vi "XYGraph_appearance.vi"() -> ()   [LabVIEW 2020]
panel:
  in  "Index Cluster":i32
  out "Array of DUT Cluster":cluster{"DUT (x)":dbl[], "DUT (y)":dbl[]}[](array[cluster])
  out "XY Graph":cluster{"DUT (x)":dbl[], "DUT (y)":dbl[]}[](graph)
  out "Display -> REFNUM : Test Voltages Results Temp Array":dbl[](array[numeric])
  out "Display -> REFNUM : Capacitance Results Temp Array":dbl[](array[numeric])
  in  "Array Size":i32
  out "Display -> GLOBAL VARIABLE : Array size(s)":i32
  in  "Test Voltages Results Temp Array":dbl[](array[numeric])
  in  "Capacitance Results Temp Array":dbl[](array[numeric])
  out "error out":errorcluster
  in  "error in (no error)":errorcluster
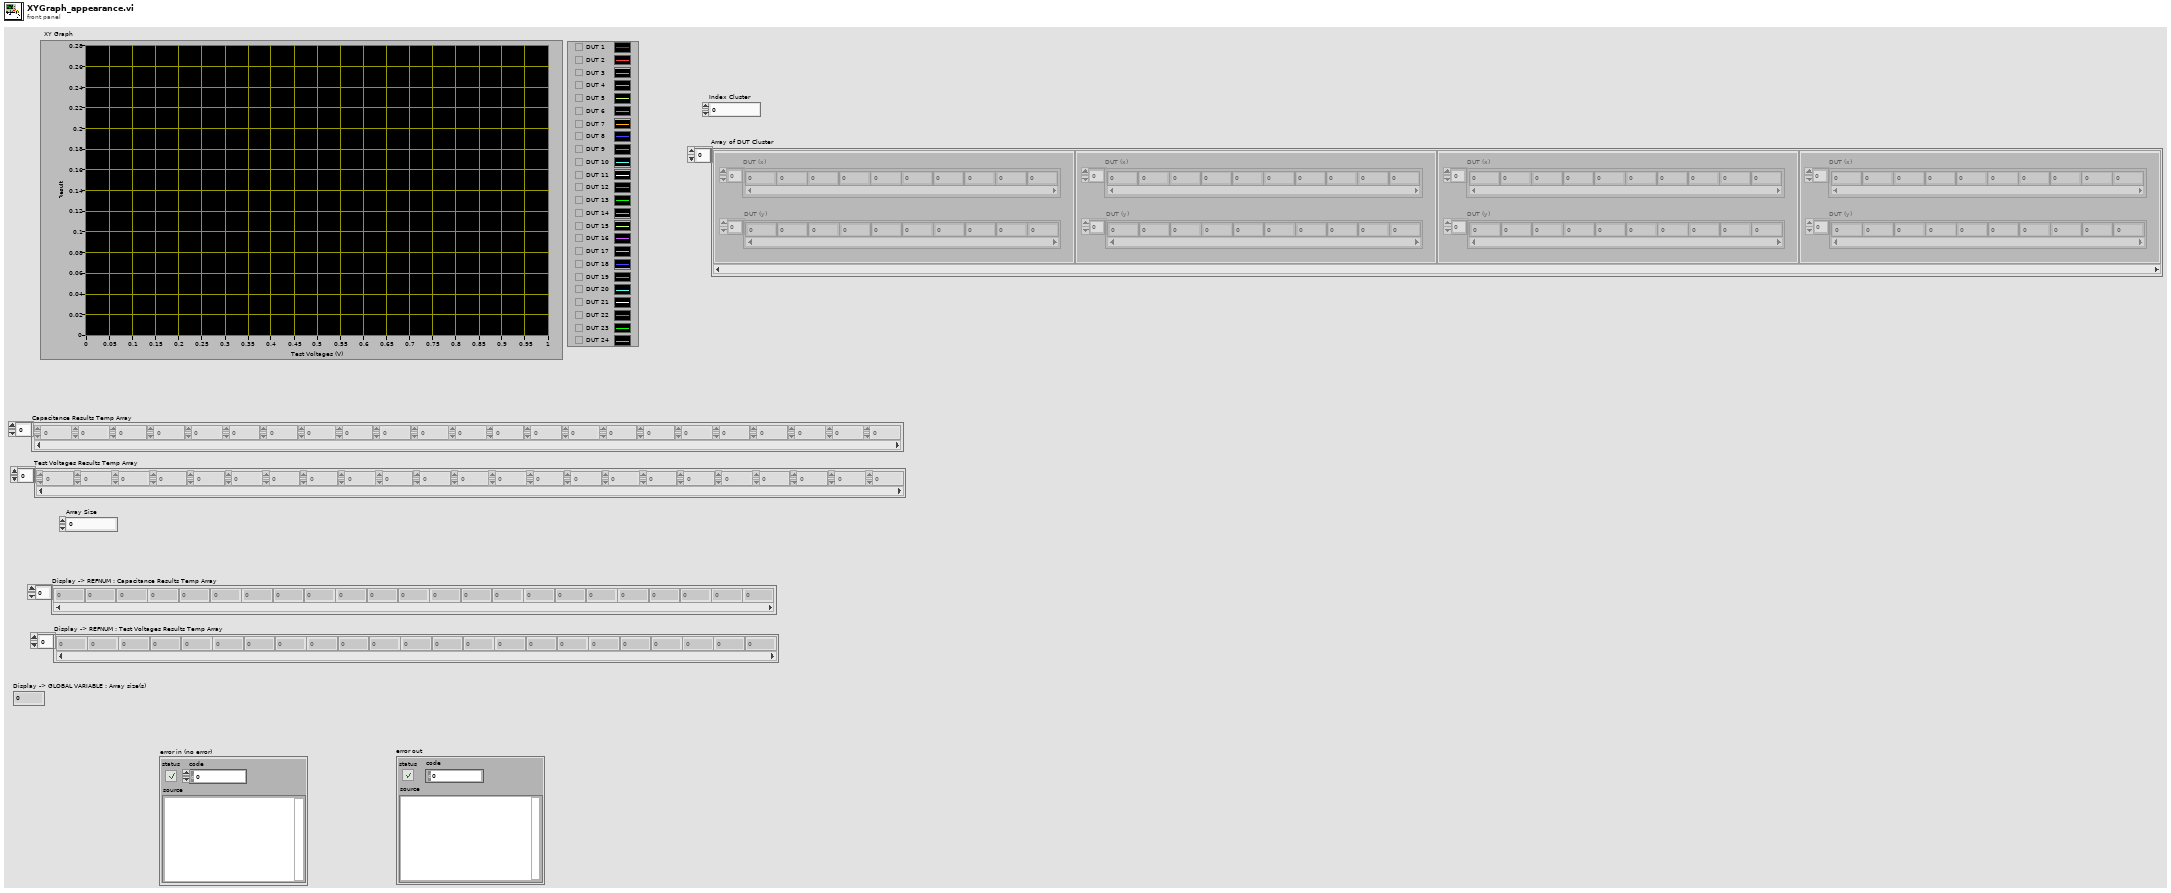
[diagram p1: front panel]
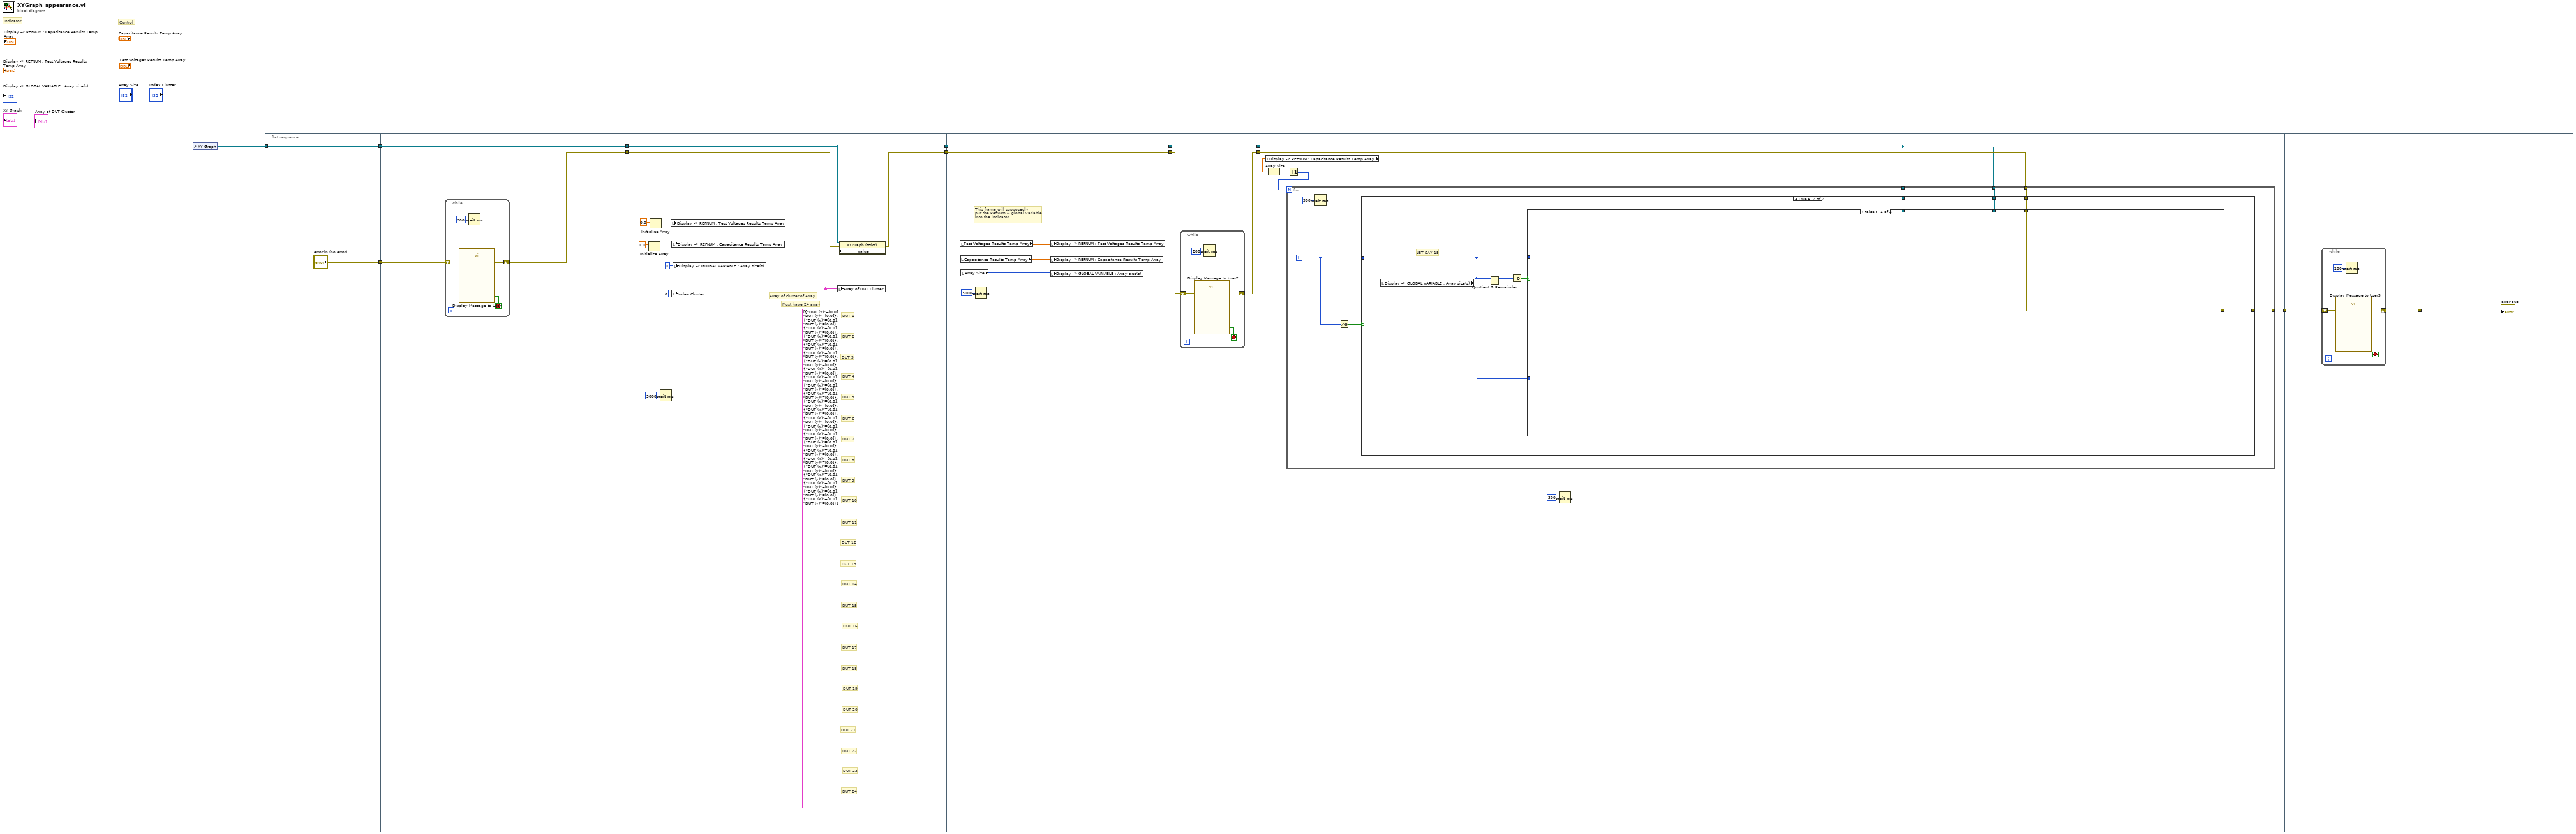
[diagram p0: block diagram]
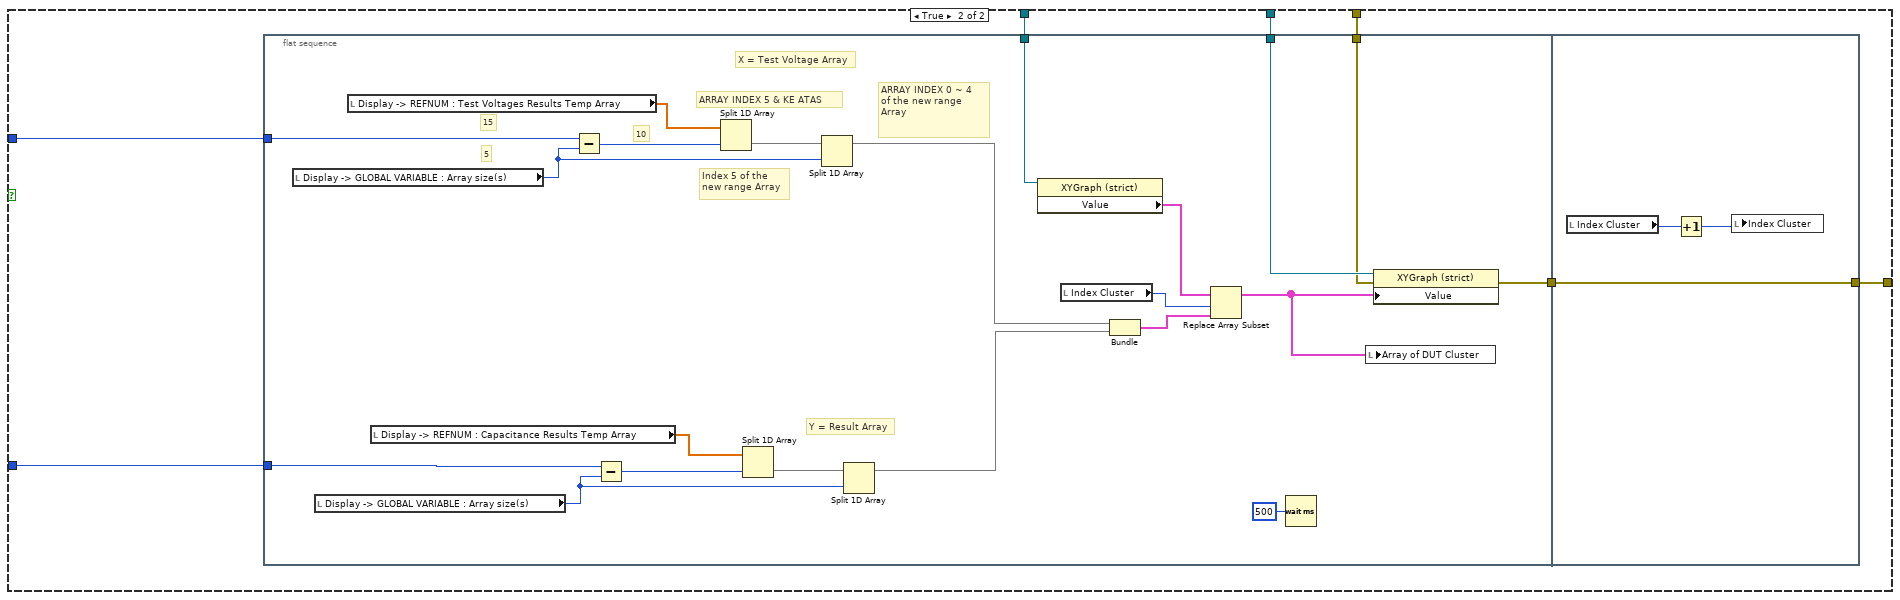
[diagram p3: hidden frame]
diagram:
  # "Indicator"
  # "Control"
  n1 = control-ref of="XY Graph"() -> (w1:refnum<vi>)
  n2 = flat-sequence {
    tunnel: w1 -> [w15]
    tunnel: [w15] -> w13
    tunnel: ["error in (no error)"] -> w12
    tunnel: [w18] -> w11
    tunnel: [w17] -> w10
    tunnel: w13 -> [w18]
    tunnel: w12 -> [w16]
    tunnel: [w27] -> w9
    tunnel: w11 -> [w27]
    tunnel: [w25] -> w8
    tunnel: w10 -> [w26]
    tunnel: [w35] -> w7
    tunnel: w9 -> [w35]
    tunnel: [w34] -> w6
    tunnel: w8 -> [w34]
    tunnel: [w42] -> w5
    tunnel: w7 -> [w42]
    tunnel: [w40] -> w4
    tunnel: w6 -> [w41]
    tunnel: w5 -> [w49]
    tunnel: w4 -> [w51]
    tunnel: [w50] -> w3
    tunnel: w3 -> [w103]
    tunnel: [w102] -> w2
    tunnel: w2 -> [w108]
    frame #0 {
    }
    frame #1 {
      n3 = while {
        shift-right: [w20] -> w17
        shift-left: w16 -> [w21]
        stop <- w19 stop-if-true
        n4 = call "Display Message to User"("error in (no error)"=w21) -> ("error out"=w20:errorcluster, "OK"=w19:bool)  [unwired: 9 in]
        n5 = Wait (ms)(milliseconds to wait=u32 200) -> ()  [unwired: 1 out]
      }
    }
    frame #2 {
      w24 = cluster{"DUT (x)":dbl[], "DUT (y)":dbl[]}[] [{"DUT (x)"=[0.0], "DUT (y)"=[0.0]}, {"DUT (x)"=[0.0], "DUT (y)"=[0.0]}, {"DUT (x)"=[0.0], "DUT (y)"=[0.0]}, {"DUT (x)"=[0.0], "DUT (y)"=[0.0]}, {"DUT (x)"=[0.0], "DUT (y)"=[0.0]}, {"DUT (x)"=[0.0], "DUT (y)"=[0.0]}, {"DUT (x)"=[0.0], "DUT (y)"=[0.0]}, {"DUT (x)"=[0.0], "DUT (y)"=[0.0]}, {"DUT (x)"=[0.0], "DUT (y)"=[0.0]}, {"DUT (x)"=[0.0], "DUT (y)"=[0.0]}, {"DUT (x)"=[0.0], "DUT (y)"=[0.0]}, {"DUT (x)"=[0.0], "DUT (y)"=[0.0]}, {"DUT (x)"=[0.0], "DUT (y)"=[0.0]}, {"DUT (x)"=[0.0], "DUT (y)"=[0.0]}, {"DUT (x)"=[0.0], "DUT (y)"=[0.0]}, {"DUT (x)"=[0.0], "DUT (y)"=[0.0]}, {"DUT (x)"=[0.0], "DUT (y)"=[0.0]}, {"DUT (x)"=[0.0], "DUT (y)"=[0.0]}, {"DUT (x)"=[0.0], "DUT (y)"=[0.0]}, {"DUT (x)"=[0.0], "DUT (y)"=[0.0]}, {"DUT (x)"=[0.0], "DUT (y)"=[0.0]}, {"DUT (x)"=[0.0], "DUT (y)"=[0.0]}, {"DUT (x)"=[0.0], "DUT (y)"=[0.0]}, {"DUT (x)"=[0.0], "DUT (y)"=[0.0]}] ("Array of DUT Cluster")
      # "DUT 24"
      # "DUT 23"
      # "DUT 22"
      # "DUT 21"
      # "DUT 20"
      # "DUT 19"
      # "DUT 18"
      # "DUT 17"
      # "DUT 16"
      # "DUT 15"
      # "DUT 14"
      # "DUT 13"
      # "DUT 12"
      # "DUT 11"
      # "DUT 10"
      # "DUT 9"
      # "DUT 8"
      # "DUT 7"
      # "DUT 6"
      # "DUT 5"
      # "DUT 4"
      # "DUT 3"
      # "DUT 2"
      # "DUT 1"
      # "Array of cluster of Array"
      # "Must have 24 array"
      n6 = Initialize Array(0.0 ("element")) -> (w29:dbl[])  [unwired: 1 in]
      n7 = Initialize Array(0.0 ("element")) -> (w30:dbl[])  [unwired: 1 in]
      n8 = Wait (ms)(milliseconds to wait=u32 3000) -> ()  [unwired: 1 out]
      n9 = local write "Display -> REFNUM : Test Voltages Results Temp Array"(w30) -> ()
      n10 = local write "Display -> REFNUM : Capacitance Results Temp Array"(w29) -> ()
      n11 = local write "Index Cluster"(0 ("Index Cluster")) -> ()
      n12 = local write "Display -> GLOBAL VARIABLE : Array size(s)"(0 ("Display -> GLOBAL VARIABLE : Array size(s)")) -> ()
      n13 = local write "Array of DUT Cluster"(w24) -> ()
      n14 = property class="XYGraph (strict)"(reference=w27, error in=w26, "Value"=w24) -> (error out=w25:errorcluster)  [unwired: 1 out]
    }
    frame #3 {
      # "This frame will supposedly \nput the RefNUm & global variable\ninto the indicator"
      n15 = local read "Test Voltages Results Temp Array"() -> (w39:dbl[])
      n16 = local read "Capacitance Results Temp Array"() -> (w38:dbl[])
      n17 = local read "Array Size"() -> (w37:i32)
      n18 = Wait (ms)(milliseconds to wait=u32 3000) -> ()  [unwired: 1 out]
      n19 = local write "Display -> REFNUM : Test Voltages Results Temp Array"(w39) -> ()
      n20 = local write "Display -> REFNUM : Capacitance Results Temp Array"(w38) -> ()
      n21 = local write "Display -> GLOBAL VARIABLE : Array size(s)"(w37) -> ()
    }
    frame #4 {
      n22 = while {
        shift-right: [w44] -> w40
        shift-left: w41 -> [w45]
        stop <- w43 stop-if-true
        n23 = call "Display Message to User2"("error in (no error)"=w45) -> ("error out"=w44:errorcluster, "OK"=w43:bool)  [unwired: 9 in]
        n24 = Wait (ms)(milliseconds to wait=u32 200) -> ()  [unwired: 1 out]
      }
    }
    frame #5 {
      n25 = local read "Display -> REFNUM : Capacitance Results Temp Array"() -> (w53:dbl[])
      n26 = Array Size(array=w53) -> (size(s)=w48:i32)
      n27 = Increment(x=w48) -> (x+1=w47:i32)
      n28 = for {
        N: w47 -> [_]
        tunnel: w49 -> [w60]
        tunnel: w51 -> [w58]
        tunnel: [w57] -> w50
        tunnel: w49 -> [w56]
        i -> [w55]
        n29 = Wait (ms)(milliseconds to wait=u32 300) -> ()  [unwired: 1 out]
        n30 = Not Equal To 0?(x=w55) -> (x != 0?=w54:bool)
        n31 = case shown="True" w54 {
          tunnel: w60 -> [_ w66]
          tunnel: w58 -> [w61 w65]
          tunnel: [w61 w64] -> w57
          tunnel: w56 -> [_ w63]
          tunnel: w55 -> [_ w62]
          frame False {
          }
          frame True {
            # "LET SAY 15"
            n32 = local read "Display -> GLOBAL VARIABLE : Array size(s)"() -> (w69:i32)
            n33 = Quotient & Remainder(x=w62, y=w69) -> (x-y*floor(x/y)=w68:i32)  [unwired: 1 out]
            n34 = Equal To 0?(x=w68) -> (x = 0?=w67:bool)
            n35 = case shown="False" w67 {
              tunnel: w62 -> [_ w77]
              tunnel: w62 -> [_ w76]
              tunnel: w66 -> [_ w75]
              tunnel: w65 -> [w70 w74]
              tunnel: [w70 w73] -> w64
              tunnel: w63 -> [_ w72]
              frame False {
              }
              frame True {
                n36 = flat-sequence {
                  tunnel: w77 -> [w80]
                  tunnel: w76 -> [w81]
                  tunnel: w75 -> [w94]
                  tunnel: w74 -> [w93]
                  tunnel: w72 -> [w89]
                  tunnel: [w92] -> w71
                  tunnel: [w101] -> w73
                  tunnel: w71 -> [w101]
                  frame #0 {
                    # "Index 5 of the\nnew range Array"
                    # "ARRAY INDEX 0 ~ 4\nof the new range Array"
                    # "ARRAY INDEX 5 & KE ATAS"
                    # "10"
                    # "5"
                    # "15"
                    # "Y = Result Array"
                    # "X = Test Voltage Array"
                    n37 = local read "Display -> GLOBAL VARIABLE : Array size(s)"() -> (w79:i32)
                    n38 = local read "Display -> GLOBAL VARIABLE : Array size(s)"() -> (w78:i32)
                    n39 = local read "Display -> REFNUM : Test Voltages Results Temp Array"() -> (w97:dbl[])
                    n40 = local read "Display -> REFNUM : Capacitance Results Temp Array"() -> (w95:dbl[])
                    n41 = Subtract(x=w80, y=w79) -> (x-y=w84:i32)
                    n42 = Subtract(x=w81, y=w78) -> (x-y=w82:i32)
                    n43 = Split 1D Array(array=w97, index=w84) -> (second subarray=w98:dbl[])  [unwired: 1 out]
                    n44 = Split 1D Array(array=w95, index=w82) -> (second subarray=w96:dbl[])  [unwired: 1 out]
                    n45 = Split 1D Array(array=w98, index=w79) -> (first subarray=w91:dbl[])  [unwired: 1 out]
                    n46 = Split 1D Array(array=w96, index=w78) -> (first subarray=w90:dbl[])  [unwired: 1 out]
                    n47 = property class="XYGraph (strict)"(reference=w89) -> ("Value"=w88:cluster{"DUT (x)":dbl[], "DUT (y)":dbl[]}[])  [unwired: 1 in, 2 out]
                    n48 = local read "Index Cluster"() -> (w85:i32)
                    n49 = Bundle(w91, w90) -> (w87:cluster{dbl[], dbl[]})  [unwired: 1 in]
                    n50 = Replace Array Subset(array=w88, new element=w87, index=w85) -> (w86:cluster{"DUT (x)":dbl[], "DUT (y)":dbl[]}[])
                    n51 = Wait (ms)(milliseconds to wait=u32 500) -> ()  [unwired: 1 out]
                    n52 = local write "Array of DUT Cluster"(w86) -> ()
                    n53 = property class="XYGraph (strict)"(reference=w94, error in=w93, "Value"=w86) -> (error out=w92:errorcluster)  [unwired: 1 out]
                  }
                  frame #1 {
                    n54 = local read "Index Cluster"() -> (w100:i32)
                    n55 = Increment(x=w100) -> (x+1=w99:i32)
                    n56 = local write "Index Cluster"(w99) -> ()
                  }
                }
              }
            }
          }
        }
      }
      n57 = Wait (ms)(milliseconds to wait=u32 300) -> ()  [unwired: 1 out]
    }
    frame #6 {
      n58 = while {
        shift-right: [w105] -> w102
        shift-left: w103 -> [w106]
        stop <- w104 stop-if-true
        n59 = call "Display Message to User3"("error in (no error)"=w106) -> ("error out"=w105:errorcluster, "OK"=w104:bool)  [unwired: 9 in]
        n60 = Wait (ms)(milliseconds to wait=u32 200) -> ()  [unwired: 1 out]
      }
    }
    frame #7 {
      "error out" <- w108
    }
  }
